vi "zadania testowe lab4.vi"() -> ()   [LabVIEW 2015]
panel:
  out "Wieksza niz 0,5":bool
  out "iteracja":i32
  out "liczba":dbl
  in  "losuj":bool
  in  "stop":bool
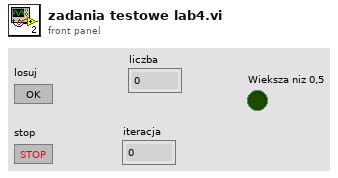
[diagram p1: front panel]
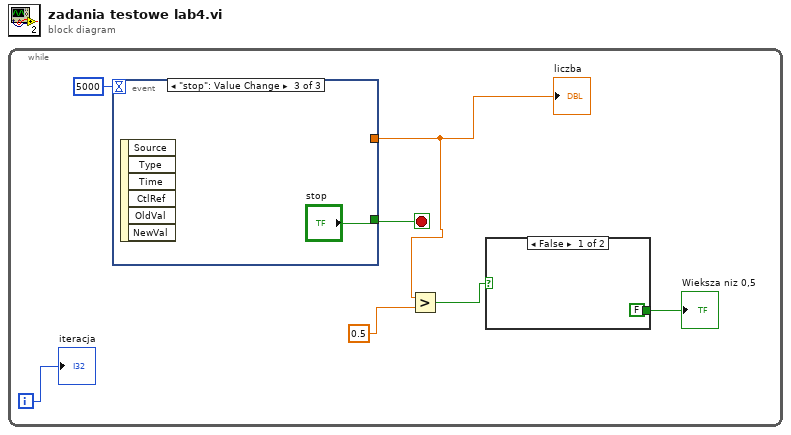
[diagram p0: block diagram]
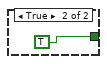
[diagram p2: hidden frame]
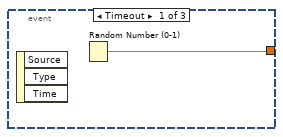
[diagram p3: hidden frame]
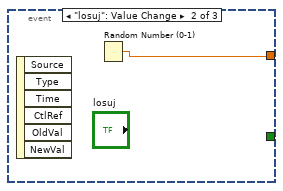
[diagram p4: hidden frame]
diagram:
  n1 = while {
    i -> [w7]
    stop <- w5 stop-if-true
    n2 = event shown="[2] \"stop\": Value Change" {
      selector: _ -> [_ _ _]
      dyn-events: _ -> [_ _ _]
      timeout: 5000 -> [_ _ _]
      tunnel: [w10 w11 _] -> w3
      tunnel: [_ _ "stop"] -> w5
      event Timeout {
        n3 = event-data() -> ()  [unwired: 1 in, 3 out]
        n4 = Random Number (0-1)() -> (number: 0 to 1=w10:dbl)
      }
      event "losuj": Value Change {
        n5 = event-data() -> ()  [unwired: 1 in, 6 out]
        n6 = Random Number (0-1)() -> (number: 0 to 1=w11:dbl)
      }
      event "stop": Value Change {
        n7 = event-data() -> ()  [unwired: 1 in, 6 out]
      }
    }
    "liczba" <- w3
    n8 = Greater?(x=w3, y=0.5) -> (0:w2:bool)
    n9 = case shown="False" w2 {
      tunnel: [FALSE ("Wieksza niz 0,5") TRUE ("Wieksza niz 0,5")] -> w1
      frame False {
      }
      frame True {
      }
    }
    "Wieksza niz 0,5" <- w1
    "iteracja" <- w7
  }
